vi "nii_read_head.vi"(8 "error in (no error)":errorcluster, 11 "file (use dialog)":path) -> (0 "error out":errorcluster, 2 "data value reference 2":refnum<data-value>, 3 "Data":T1 {"slice orientation" items=["transverse unflipped", "coronal unflipped", "sagittal unflipped", "transverse flipped", "coronal flipped", "sagittal flipped"]}, 4 "non-flip":bool, 5 "head":u8[](array[numeric]) format="%.0x")   [LabVIEW 2014]
uses:
  control/head_data.ctl
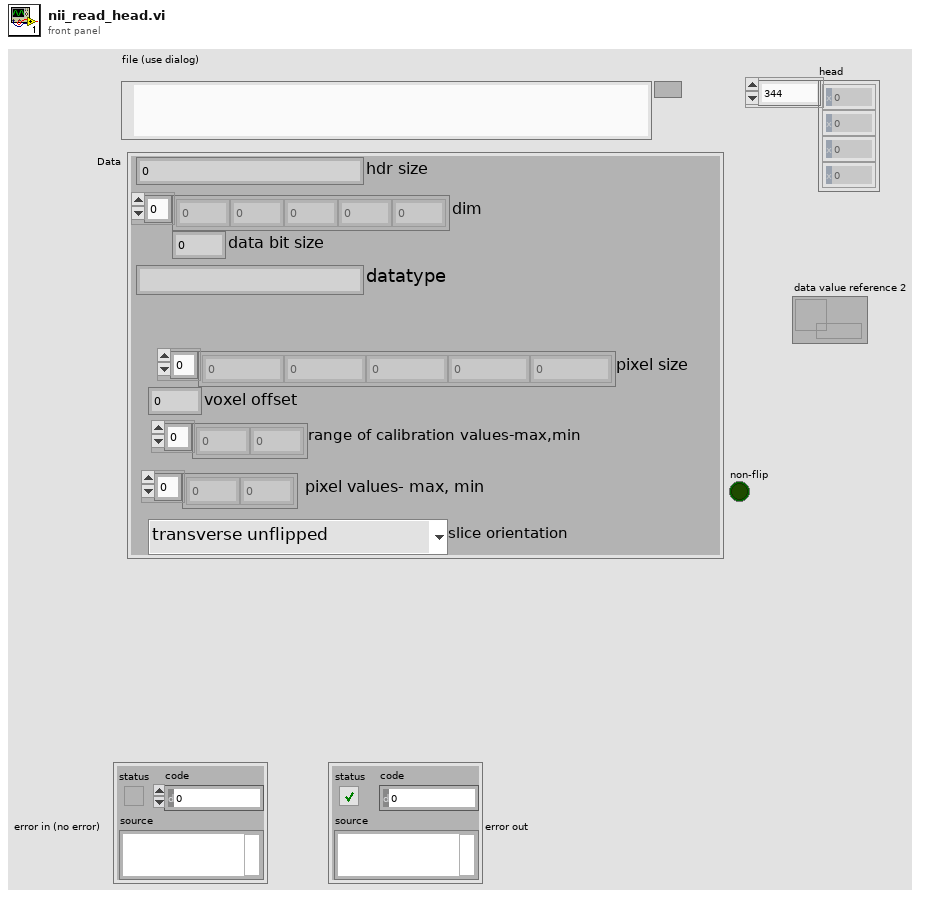
[diagram p1: front panel]
types:
  T1 = typedef "head_data.ctl" = cluster{"hdr size":i32, "dim":i32[], "data bit size":i32, "datatype":string, "pixel size ":sgl[], "voxel offset":sgl, "range of calibration values-max,min":sgl[], " pixel values- max, min":sgl[], "slice orientation":u16}
  T2 = enum16{"u_int8", "int8", "u_int16", "int16", "u_int32", "int32", "u_int64", "int64", "float", "double"}
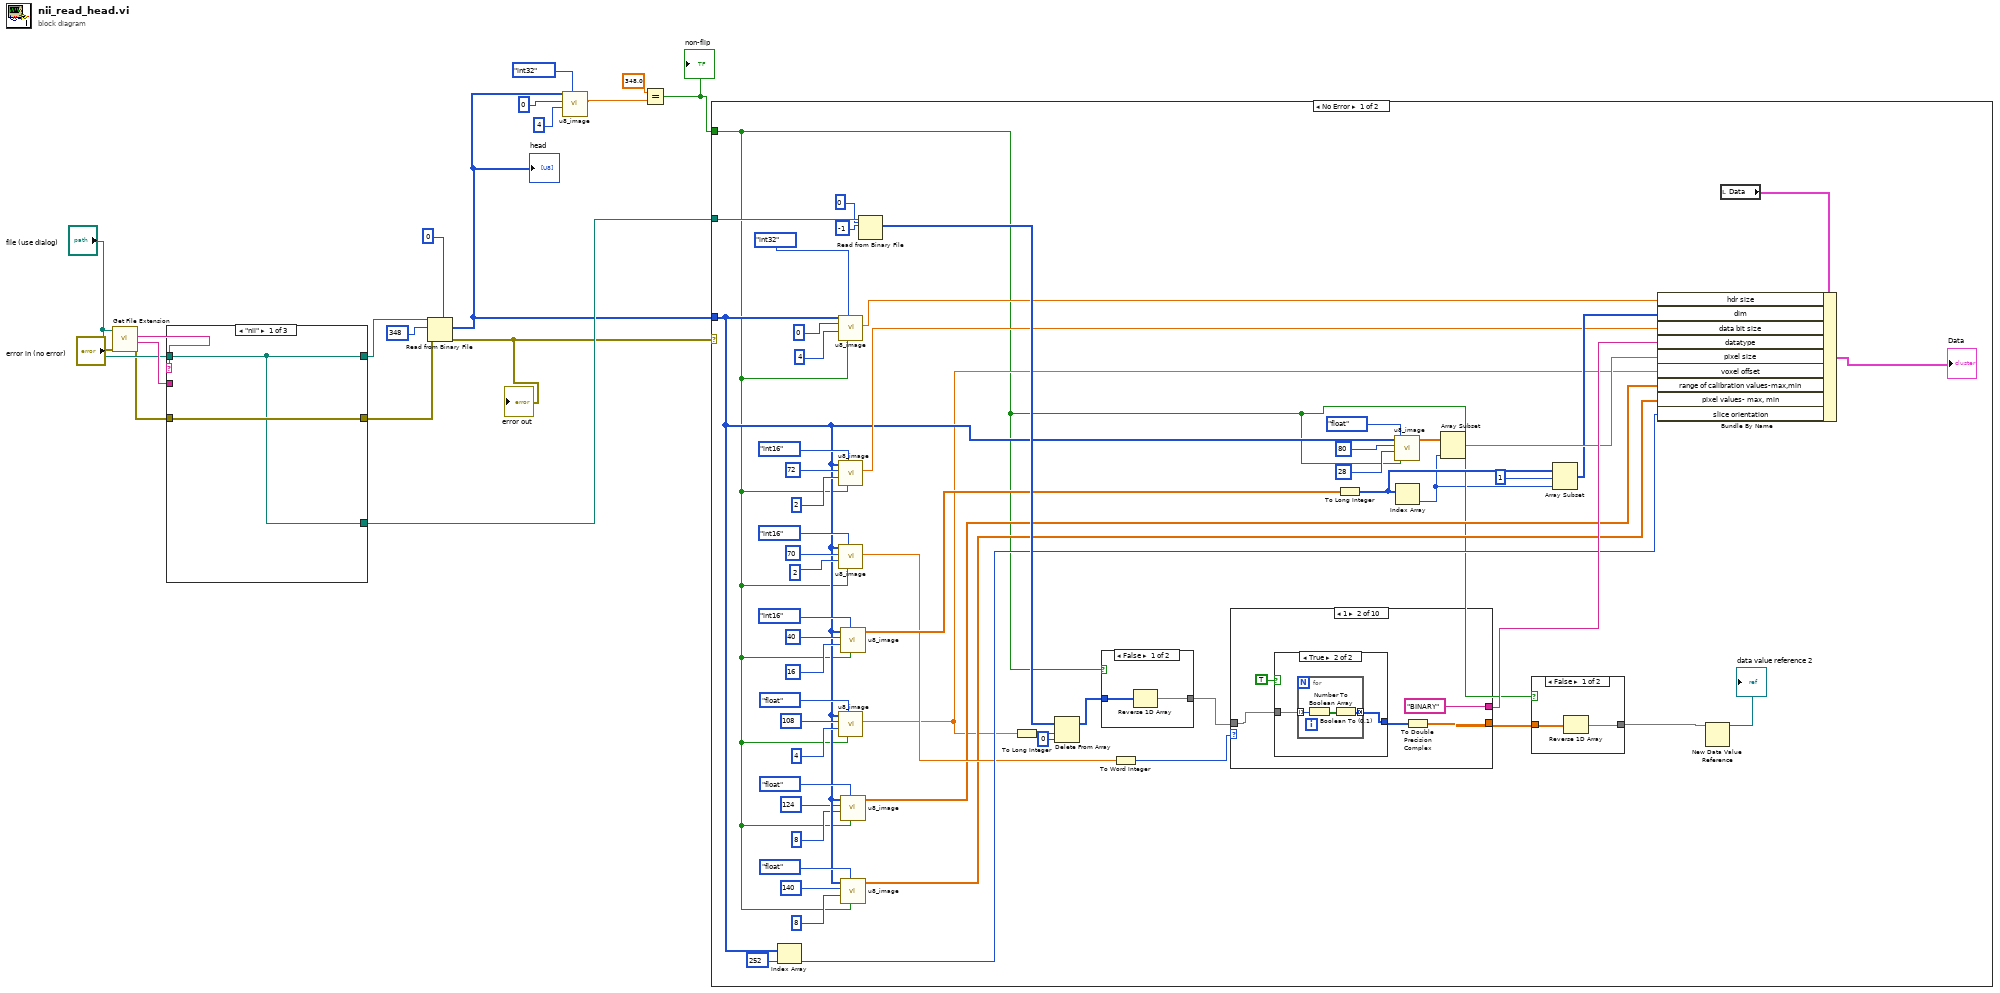
[diagram p0: block diagram]
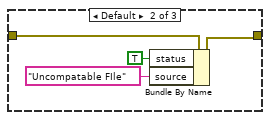
[diagram p2: hidden frame]
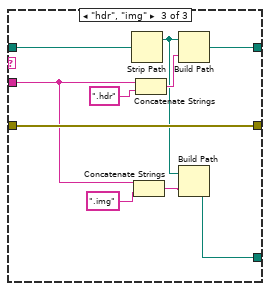
[diagram p3: hidden frame]
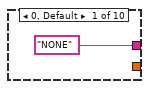
[diagram p6: hidden frame]
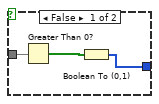
[diagram p7: hidden frame]
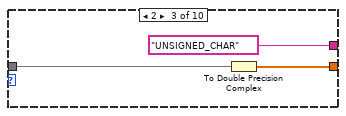
[diagram p8: hidden frame]
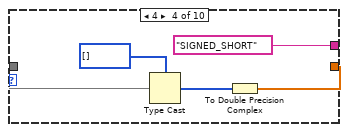
[diagram p9: hidden frame]
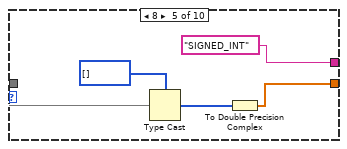
[diagram p10: hidden frame]
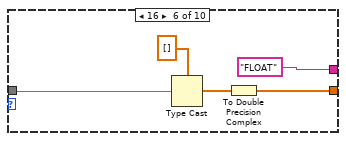
[diagram p11: hidden frame]
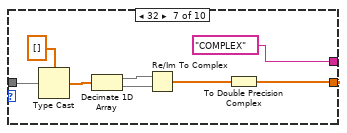
[diagram p12: hidden frame]
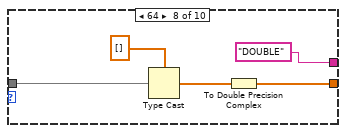
[diagram p13: hidden frame]
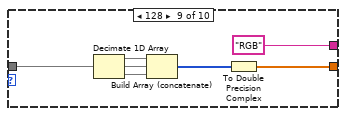
[diagram p14: hidden frame]
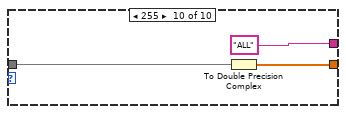
[diagram p15: hidden frame]
diagram:
  n1 = call <vilib>:"Get File Extension.vi"("error in (no error)"="error in (no error)", "file"="file (use dialog)") -> ("error out"=w14:errorcluster, "filename without extension"=w17:string, "lowercase file extension"=w18:string)  [unwired: 6 in, 1 out]
  n2 = case shown="\"nii\"" w18 {
    tunnel: "file (use dialog)" -> [w19 _ w30]
    tunnel: [w19 _ w32] -> w10
    tunnel: w17 -> [_ _ w26]
    tunnel: [w20 w23 w31] -> w15
    tunnel: w14 -> [w20 w24 w31]
    tunnel: [w19 _ w25] -> w12
    frame "nii" {
    }
    frame Default {
      n3 = Bundle By Name(cluster=w24, "status"=TRUE, "source"="Uncompatable FIle") -> (w23:errorcluster)
    }
    frame "hdr", "img" {
      n4 = Strip Path(path=w30) -> (stripped path=w29:path)  [unwired: 1 out]
      n5 = Concatenate Strings(w26, ".img" ("string")) -> (w28:string)
      n6 = Concatenate Strings(w26, ".hdr" ("string")) -> (w33:string)
      n7 = Build Path(base path=w29, name or relative path=w33) -> (appended path=w32:path)
      n8 = Build Path(base path=w29, name or relative path=w28) -> (appended path=w25:path)
    }
  }
  n9 = Read from Binary File(5:u8 0, 8:w15, 10:348 ("count (1)"), 11:w10) -> (0:w9:errorcluster, 2:w5:u8[])  [unwired: 2 in, 2 out]
  "error out" <- w9
  "head" <- w5
  n10 = call "u8_image.vi"("Enum"=T2."int32", "length"=4, "index"=0, "array"=w5) -> ("Numeric"=w3:dbl)  [unwired: 6 in, 1 out]
  n11 = Equal?(x=348.0, y=w3) -> (x = y?=w6:bool)
  "non-flip" <- w6
  n12 = case shown="No Error" w9 {
    tunnel: w5 -> [w48 _]
    tunnel: w12 -> [w90 _]
    tunnel: w6 -> [w39 _]
    frame No Error {
      n13 = Index Array(array=w48, index=252) -> (element=w82:u8)
      n14 = call "u8_image.vi"("non-flip"=w39, "Enum"=T2."int32", "length"=4, "index"=0, "array"=w48) -> ("Numeric"=w76:dbl)  [unwired: 5 in, 1 out]
      n15 = call "u8_image.vi"("non-flip"=w39, "Enum"=T2."int16", "length"=2, "index"=72, "array"=w48) -> ("Numeric"=w67:dbl)  [unwired: 5 in, 1 out]
      n16 = call "u8_image.vi"("non-flip"=w39, "Enum"=T2."int16", "length"=2, "index"=70, "array"=w48) -> ("Numeric"=w63:dbl)  [unwired: 5 in, 1 out]
      n17 = call "u8_image.vi"("non-flip"=w39, "Enum"=T2."float", "length"=4, "index"=108, "array"=w48) -> ("Numeric"=w45:dbl)  [unwired: 5 in, 1 out]
      n18 = call "u8_image.vi"("non-flip"=w39, "Enum"=T2."int16", "length"=16, "index"=40, "array"=w48) -> ("Array"=w73:dbl[])  [unwired: 5 in, 1 out]
      n19 = call "u8_image.vi"("non-flip"=w39, "Enum"=T2."float", "length"=8, "index"=124, "array"=w48) -> ("Array"=w49:dbl[])  [unwired: 5 in, 1 out]
      n20 = call "u8_image.vi"("non-flip"=w39, "Enum"=T2."float", "length"=8, "index"=140, "array"=w48) -> ("Array"=w52:dbl[])  [unwired: 5 in, 1 out]
      n21 = Read from Binary File(5:u8 0 ("default value 1"), 10:-1 ("count (1)"), 11:w90) -> (2:w87:u8[])  [unwired: 3 in, 3 out]
      n22 = To Long Integer(number=w45) -> (32bit integer=w44:i32)
      n23 = Delete From Array(array=w87, length=w44, index=0) -> (array with subset deleted=w42:u8[])  [unwired: 1 out]
      n24 = case shown="False" w39 {
        tunnel: [w94 w96] -> w41
        tunnel: w42 -> [w95 w96]
        frame False {
          n25 = Reverse 1D Array(array=w95) -> (reversed array=w94:u8[])
        }
        frame True {
        }
      }
      n26 = To Word Integer(number=w63) -> (16bit integer=w62:i16)
      n27 = case shown="1" w62 {
        tunnel: ["NONE" "BINARY" "UNSIGNED_CHAR" "SIGNED_SHORT" "SIGNED_INT" "FLOAT" "COMPLEX" "DOUBLE" "RGB" "ALL"] -> w86
        tunnel: [_ w101 w112 w117 w122 w127 w132 w140 w143 w149] -> w40
        tunnel: w41 -> [_ w99 w111 w116 w120 w124 w129 w137 w144 w150]
        frame 0, Default {
        }
        frame 1 {
          n28 = case shown="True" TRUE {
            tunnel: w99 -> [w104 w107]
            tunnel: [w103 w106] -> w100
            frame False {
              n29 = Greater Than 0?(x=w104) -> (x > 0?=w105:bool[])
              n30 = Boolean To (0,1)(Boolean=w105) -> (0, 1=w103:i16[])
            }
            frame True {
              n31 = for {
                tunnel: w107 -> [w110] mode=indexing
                tunnel: [w108] -> w106 mode=concatenating
                n32 = Number To Boolean Array(number=w110) -> (Boolean array=w109:bool[])
                n33 = Boolean To (0,1)(Boolean=w109) -> (0, 1=w108:i16[])
              }
            }
          }
          n34 = To Double Precision Complex(1:w100) -> (0:w101:cdb[])
        }
        frame 2 {
          n35 = To Double Precision Complex(1:w111) -> (0:w112:cdb[])
        }
        frame 4 {
          n36 = Type Cast(type=i16[] [], x=w116) -> (*(type *) &x=w115:i16[])
          n37 = To Double Precision Complex(1:w115) -> (0:w117:cdb[])
        }
        frame 8 {
          n38 = Type Cast(type=i32[] [], x=w120) -> (*(type *) &x=w119:i32[])
          n39 = To Double Precision Complex(1:w119) -> (0:w122:cdb[])
        }
        frame 16 {
          n40 = Type Cast(type=sgl[] [], x=w124) -> (*(type *) &x=w125:sgl[])
          n41 = To Double Precision Complex(1:w125) -> (0:w127:cdb[])
        }
        frame 32 {
          n42 = Type Cast(type=sgl[] [], x=w129) -> (*(type *) &x=w130:sgl[])
          n43 = Decimate 1D Array(w130) -> (w135:sgl[], w134:sgl[])
          n44 = Re/Im To Complex(1:w134, 2:w135) -> (0:w133:csg[])
          n45 = To Double Precision Complex(1:w133) -> (0:w132:cdb[])
        }
        frame 64 {
          n46 = Type Cast(type=dbl[] [], x=w137) -> (*(type *) &x=w138:dbl[])
          n47 = To Double Precision Complex(1:w138) -> (0:w140:cdb[])
        }
        frame 128 {
          n48 = Decimate 1D Array(w144) -> (w147:u8[], w146:u8[], w145:u8[])
          n49 = Build Array (concatenate)(w147, w146, w145) -> (w142:u8[])
          n50 = To Double Precision Complex(1:w142) -> (0:w143:cdb[])
        }
        frame 255 {
          n51 = To Double Precision Complex(1:w150) -> (0:w149:cdb[])
        }
      }
      n52 = To Long Integer(number=w73) -> (32bit integer=w79:i32[])
      n53 = call "u8_image.vi"("non-flip"=w39, "Enum"=T2."float", "length"=28, "index"=80, "array"=w48) -> ("Array"=w59:dbl[])  [unwired: 5 in, 1 out]
      n54 = Index Array(array=w79) -> (element=w38:i32)  [unwired: 1 in]
      n55 = Array Subset(array=w59, length=w38) -> (w85:dbl[])  [unwired: 1 in]
      n56 = case shown="False" w39 {
        tunnel: [w91 w93] -> w36
        tunnel: w40 -> [w92 w93]
        frame False {
          n57 = Reverse 1D Array(array=w92) -> (reversed array=w91:cdb[])
        }
        frame True {
        }
      }
      n58 = Array Subset(array=w79, index=1, length=w38) -> (w80:i32[])
      n59 = New Data Value Reference(data value=w36) -> (data value reference=→"data value reference 2":refnum<data-value>)  [unwired: 1 in, 1 out]
      n60 = local read "Data"() -> (w84:T1)
      n61 = Bundle By Name(cluster=w84, "hdr size"=w76, "dim"=w80, "data bit size"=w67, "datatype"=w86, "pixel size"=w85, "voxel offset"=w45, "range of calibration values-max,min"=w49, "pixel values- max, min"=w52, "slice orientation"=w82) -> (→"Data":T1)
    }
    frame Error {
    }
  }
